vi "ESC_StdSci_WorkBench_fnl.vi"() -> ()   [LabVIEW 2015]
uses:
  SCI_DataPck.ctl
  SCI_DataType.ctl
panel:
  out "串口读缓存字符数":u32
  in  "VISA资源名称":refnum<visa-resource-name>="COM1"
  out "串口读数据":i32[](array[numeric]) format="%04x"
  out "串口缓存非空":bool
  out "串口写入数据":string
  out "串口读数据包":T1={"包头"=170, "数据低8位"=0, "数据低高8位"=0, "数据类型"=0, "CRC余数"=0, "数据无效"=FALSE, "数据更新"=FALSE} {"包头" format="%02x"; "数据低8位" format="%02x"; "数据低高8位" format="%02x"; "数据类型" items=["VOID"]; "CRC余数" format="%02x"}
  out "串口预写入簇":T1={"包头"=170, "数据低8位"=0, "数据低高8位"=0, "数据类型"=0, "CRC余数"=0, "数据无效"=FALSE, "数据更新"=FALSE} {"包头" format="%02x"; "数据低8位" format="%02x"; "数据低高8位" format="%02x"; "数据类型" items=["VOID"]; "CRC余数" format="%02x"}
  out "写数据更新":bool
  in  "串口写数据包":T1={"包头"=170, "数据低8位"=0, "数据低高8位"=0, "数据类型"=0, "CRC余数"=0, "数据无效"=FALSE, "数据更新"=FALSE} {"包头" format="%02x"; "数据低8位" format="%02x"; "数据低高8位" format="%02x"; "数据类型" items=["VOID"]; "CRC余数" format="%02x"}
  in  "写入数据 2":u16 format="%x"
  in  "写入数据类型 2":u16 format="%x"
  in  "发送 2":bool
  out "写数据CRC余数 2":u16 format="%x"
  in  "停止按钮":bool
  in  "读出数据类型":u16=16 format="%02x"
  out "读数据CRC余数":u16 format="%x"
  out "读出数据":u16 format="%x"
  out "包头":u16 format="%x"
  in  "写入数据 1":u16 format="%x"
  in  "写入数据类型 1":u16 format="%x"
  in  "发送 1":bool
  out "写数据CRC余数 1":u16 format="%x"
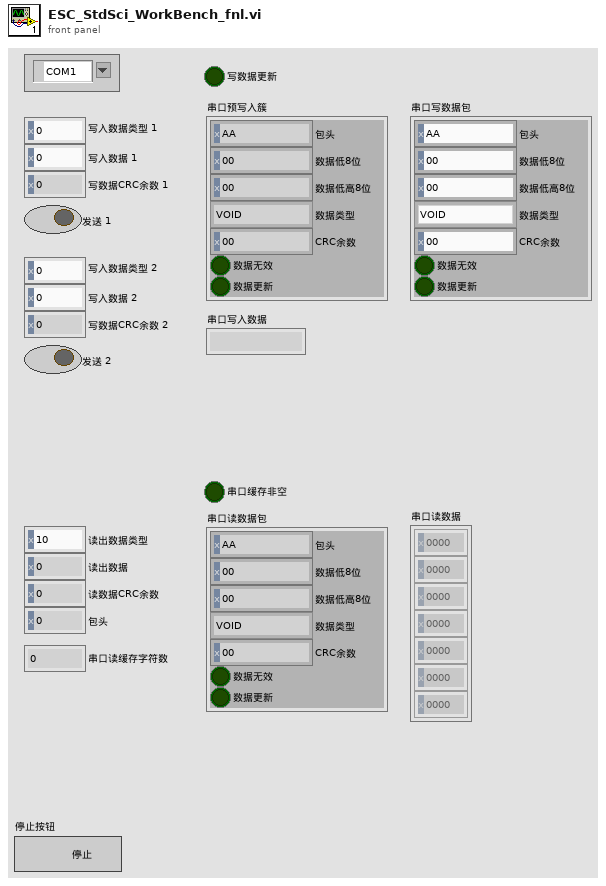
[diagram p1: front panel]
types:
  T1 = typedef "SCI_DataPck.ctl" = cluster{"包头":u16, "数据低8位":u16, "数据低高8位":u16, "数据类型":T2, "CRC余数":u16, "数据无效":bool, "数据更新":bool}
  T2 = typedef "SCI_DataType.ctl" = u16
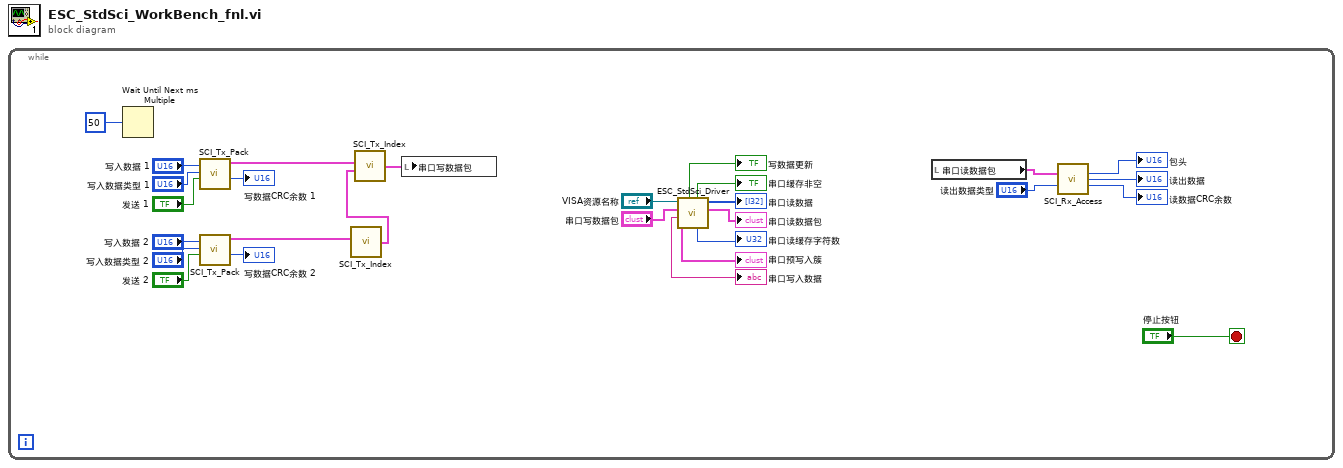
[diagram p0: block diagram]
diagram:
  n1 = while {
    stop <- "停止按钮" stop-if-true
    n2 = Wait Until Next ms Multiple(millisecond multiple=50) -> ()  [unwired: 1 out]
    n3 = call "SCI_Tx_Pack.vi"("数据有效"="发送 1", "数据类型"="写入数据类型 1", "数据"="写入数据 1") -> ("CRC余数"=→"写数据CRC余数 1":u16, "数据包输出"=w5:T1)  [unwired: 7 in]
    n4 = call "SCI_Tx_Pack.vi"("数据有效"="发送 2", "数据类型"="写入数据类型 2", "数据"="写入数据 2") -> ("CRC余数"=→"写数据CRC余数 2":u16, "数据包输出"=w6:T1)  [unwired: 7 in]
    n5 = call "SCI_Tx_Index.vi"("输入数据包（簇）"=w6) -> ("上一个包数据（簇）"=w3:T1)  [unwired: 6 in]
    n6 = call "SCI_Tx_Index.vi"("输入数据包（簇）"=w5, "下一包数据（簇）"=w3) -> ("上一个包数据（簇）"=w4:T1)  [unwired: 5 in]
    n7 = local write "串口写数据包"(w4) -> ()
    n8 = call "ESC_StdSci_Driver.vi"("串口写数据包"="串口写数据包", "VISA资源名称"="VISA资源名称") -> ("串口读数据包"=→"串口读数据包":T1, "串口读数据"=→"串口读数据":i32[], "串口读缓存字符数"=→"串口读缓存字符数":u32, "串口缓存非空"=→"串口缓存非空":bool, "写数据更新"=→"写数据更新":bool, "串口写入数据包"=→"串口预写入簇":T1, "串口写入数据"=→"串口写入数据":string)  [unwired: 3 in]
    n9 = local read "串口读数据包"() -> (w16:T1)
    n10 = call "SCI_Rx_Access.vi"("串口读数据包（簇）"=w16, "数据类型"="读出数据类型") -> ("包头"=→"包头":u16, "数据输出"=→"读出数据":u16, "CRC余数"=→"读数据CRC余数":u16)  [unwired: 11 in]
  }
